vi "VITester Toolbar Icon Paths.vi"() -> (0 "Add New TestSuite toolbar icon":path, 1 "Add New TestCase toolbar icon":path, 2 "Run All Tests toolbar icon":path, 3 "Open VI Tester toolbar icon":path)   [LabVIEW 2013]
uses:
  <userlib>/_OpenG.lib/file/file.llb/Convert File Extension (String)__ogtk.vi
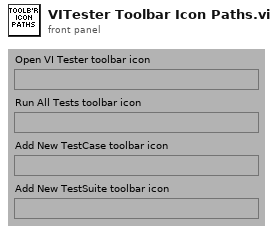
[diagram p1: front panel]
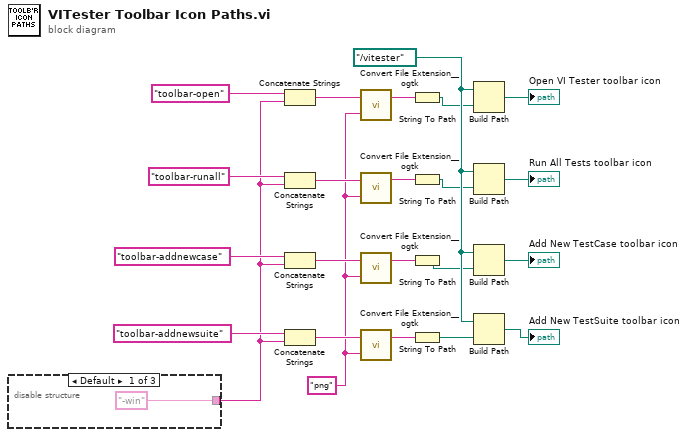
[diagram p0: block diagram]
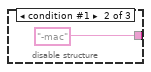
[diagram p2: hidden frame]
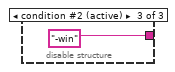
[diagram p3: hidden frame]
diagram:
  w4 = path "../vitester" ("Open VI Tester toolbar icon")
  w14 = "png" ("new ending (none)")
  n1 = disable-structure shown="Default" {
    disable-tunnel: ["-win" ("Icon File Name") "-mac" ("Icon File Name") "-win" ("Icon File Name")] -> w10
    frame condition #0 {
    }
    frame condition #1 {
    }
    frame condition #2 (active) {
    }
  }
  n2 = Concatenate Strings("toolbar-open" ("Icon File Name"), w10) -> (w22:string)
  n3 = Concatenate Strings("toolbar-runall" ("Icon File Name"), w10) -> (w18:string)
  n4 = Concatenate Strings("toolbar-addnewcase" ("Icon File Name"), w10) -> (w19:string)
  n5 = Concatenate Strings("toolbar-addnewsuite" ("Icon File Name"), w10) -> (w20:string)
  n6 = call-poly <userlib>:"Convert File Extension__ogtk.vi"("new ending (none)"=w14, "file name"=w22) -> ("new filename"=w21:string)  [unwired: 1 out]
  n7 = call-poly <userlib>:"Convert File Extension__ogtk.vi"("new ending (none)"=w14, "file name"=w18) -> ("new filename"=w11:string)  [unwired: 1 out]
  n8 = call-poly <userlib>:"Convert File Extension__ogtk.vi"("new ending (none)"=w14, "file name"=w19) -> ("new filename"=w12:string)  [unwired: 1 out]
  n9 = call-poly <userlib>:"Convert File Extension__ogtk.vi"("new ending (none)"=w14, "file name"=w20) -> ("new filename"=w13:string)  [unwired: 1 out]
  n10 = String To Path(string=w21) -> (path=w1:path)
  n11 = String To Path(string=w11) -> (path=w2:path)
  n12 = String To Path(string=w12) -> (path=w3:path)
  n13 = String To Path(string=w13) -> (path=w8:path)
  n14 = Build Path(base path=w4, name or relative path=w1) -> (appended path=→"Open VI Tester toolbar icon":path)
  n15 = Build Path(base path=w4, name or relative path=w2) -> (appended path=→"Run All Tests toolbar icon":path)
  n16 = Build Path(base path=w4, name or relative path=w3) -> (appended path=→"Add New TestCase toolbar icon":path)
  n17 = Build Path(base path=w4, name or relative path=w8) -> (appended path=→"Add New TestSuite toolbar icon":path)
